vi "Fix Column Header.vi"(1 "Numeric":i32, 2 "Titles In":string[](array[string])) -> (0 "Titles Out":string[](array[string]))   [LabVIEW 2019]
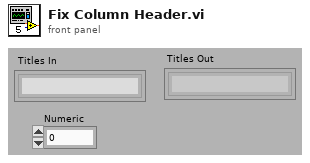
[diagram p1: front panel]
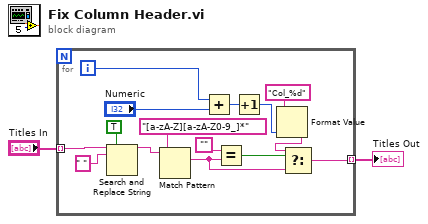
[diagram p0: block diagram]
diagram:
  n1 = for {
    tunnel: "Titles In" -> [w8] mode=indexing
    tunnel: [w5] -> w1 mode=indexing
    i -> [w3]
    n2 = Search and Replace String(replace all?=TRUE ("replace all? (F)"), input string=w8, search string=" ") -> (result string=w9:string)  [unwired: 5 in, 3 out]
    n3 = Match Pattern(string=w9, regular expression="[a-zA-Z][a-zA-Z0-9_]*") -> (match substring=w11:string)  [unwired: 1 in, 3 out]
    n4 = Add(x=w3, y="Numeric") -> (x+y=w4:i32)
    n5 = Equal?(x="", y=w11) -> (x = y?=w13:bool)
    n6 = Increment(x=w4) -> (x+1=w17:i32)
    n7 = Format Value(format string="Col_%d", value (0)=w17) -> (output string=w14:string)  [unwired: 1 in]
    n8 = Select(t=w14, s=w13, f=w11) -> (s? t:f=w5:string)
  }
  "Titles Out" <- w1
